vi "PrintLabel.vi"(6 "Print":bool, 7 "printer name (default)":string, 8 "Fixture_Data":u16[](array[numeric]), 11 "OPC_Model Type":u16 format="%x") -> ()   [LabVIEW 2017]
uses:
  <vilib>/Utility/NIReport.llb/Append Report Text (str wrap).vi
  <vilib>/Utility/NIReport.llb/NI_report.lvclass
panel:
  out "Even 2.5":string=" RR         "
  out "Line":string="KB E127652 191121SD1 0123 17:25"
  in  "margins (1.00)":T1={"top"=0.15, "left"=0.01, "right"=0.001, "bottom"=0.001} {"right" format="%.2f"; "bottom" format="%.2f"; "top" format="%.2f"; "left" format="%.2f"}
  out "Header":string="KB E127652 191121SD1 0123 17:25"
  out "Even 1.1":string=">MEGA     "
  out "Even 1.2":string=">PAD        "
  out "Even 1.3":string=" PIN       "
  out "Even 1.4":string=" WDW       "
  out "Even 1.5":string=" DL            "
  out "Even 2.1":string=" FR         "
  out "Even 2.2":string=">FL           "
  out "Even 2.3":string=">RL           "
  out "Even 2.4":string=" RR         "
  # "00 Product Number"
  # "10 Lane Number"
  # "20 Laser Number"
  # "21 Laser Number"
  # "30 Fixture Result"
  # "40 Master Unit"
  # "60 Mega Test"
  # "70 Windows Lock Press"
  # "71 Windows Lock Unpress"
  # "80 Door Lock"
  # "81 Door Unlock"
  # "90 FR Man Up"
  # "91 FR Man Down"
  # "92 FR Auto Up"
  # "93 FR Auto Down"
  # "100 RR Man Up"
  # "101 RR Man Down"
  # "110 FL Man Up"
  # "111 FL Man Down"
  # "112 FL Auto Up"
  # "113 FL  Down"
  # "120 RL Man Up"
  # "121 RL Man Down"
  # "130 LIN DR Up Contact"
  # "131 LIN DR Down Contact"
  # "132 LIN DR Auto Status"
  # "133 LIN AS Up Contact"
  # "134 LIN AS Down Contact"
  # "135 LIN AS Auto Status"
  # "136 WDW Lock Status"
  # "140 Vision Illumination"
  # "150 Vision Pin"
  # "160 QR Code Reader"
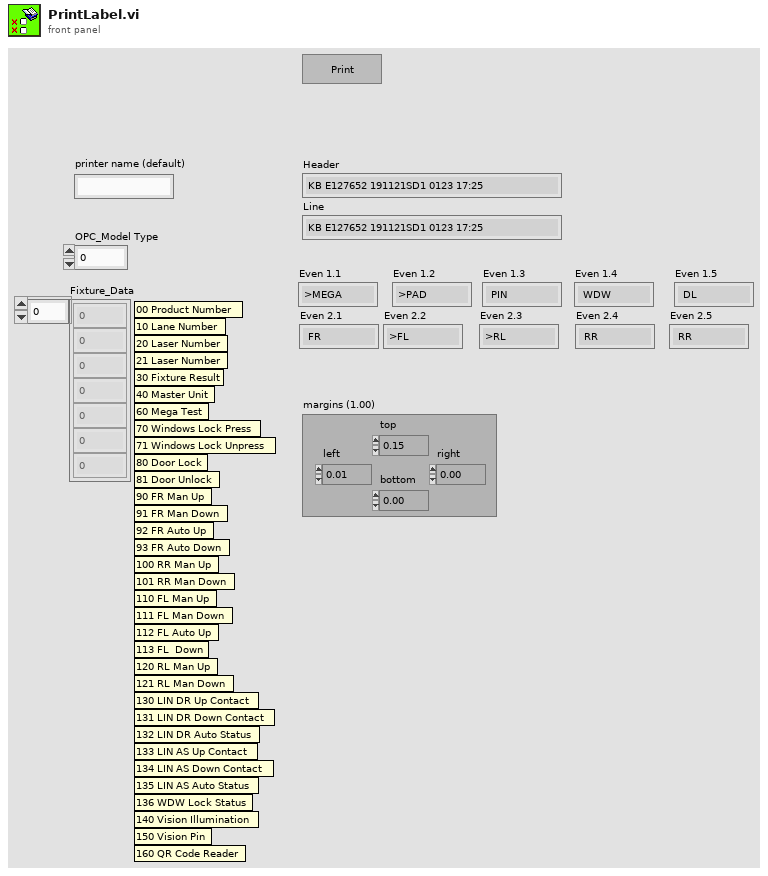
[diagram p1: front panel]
types:
  T1 = cluster{"top":dbl, "left":dbl, "right":dbl, "bottom":dbl}
  T2 = cluster{"Italic":enum16{"Italic Unchanged", "Italic On", "Italic Off"}, "Strike Through":enum16{"Strike Through Unchanged", "Strike Through On", "Strike Through Off"}, "Underline":enum16{"Underline Unchanged", "Underline On", "Underline Off"}, "Bold":enum16{"Bold Unchanged", "Bold On", "Bold Off"}}
  T3 = cluster{"Charset (-1)":i16, "Weight (-1)":i16, "Name":string, "Size":string}
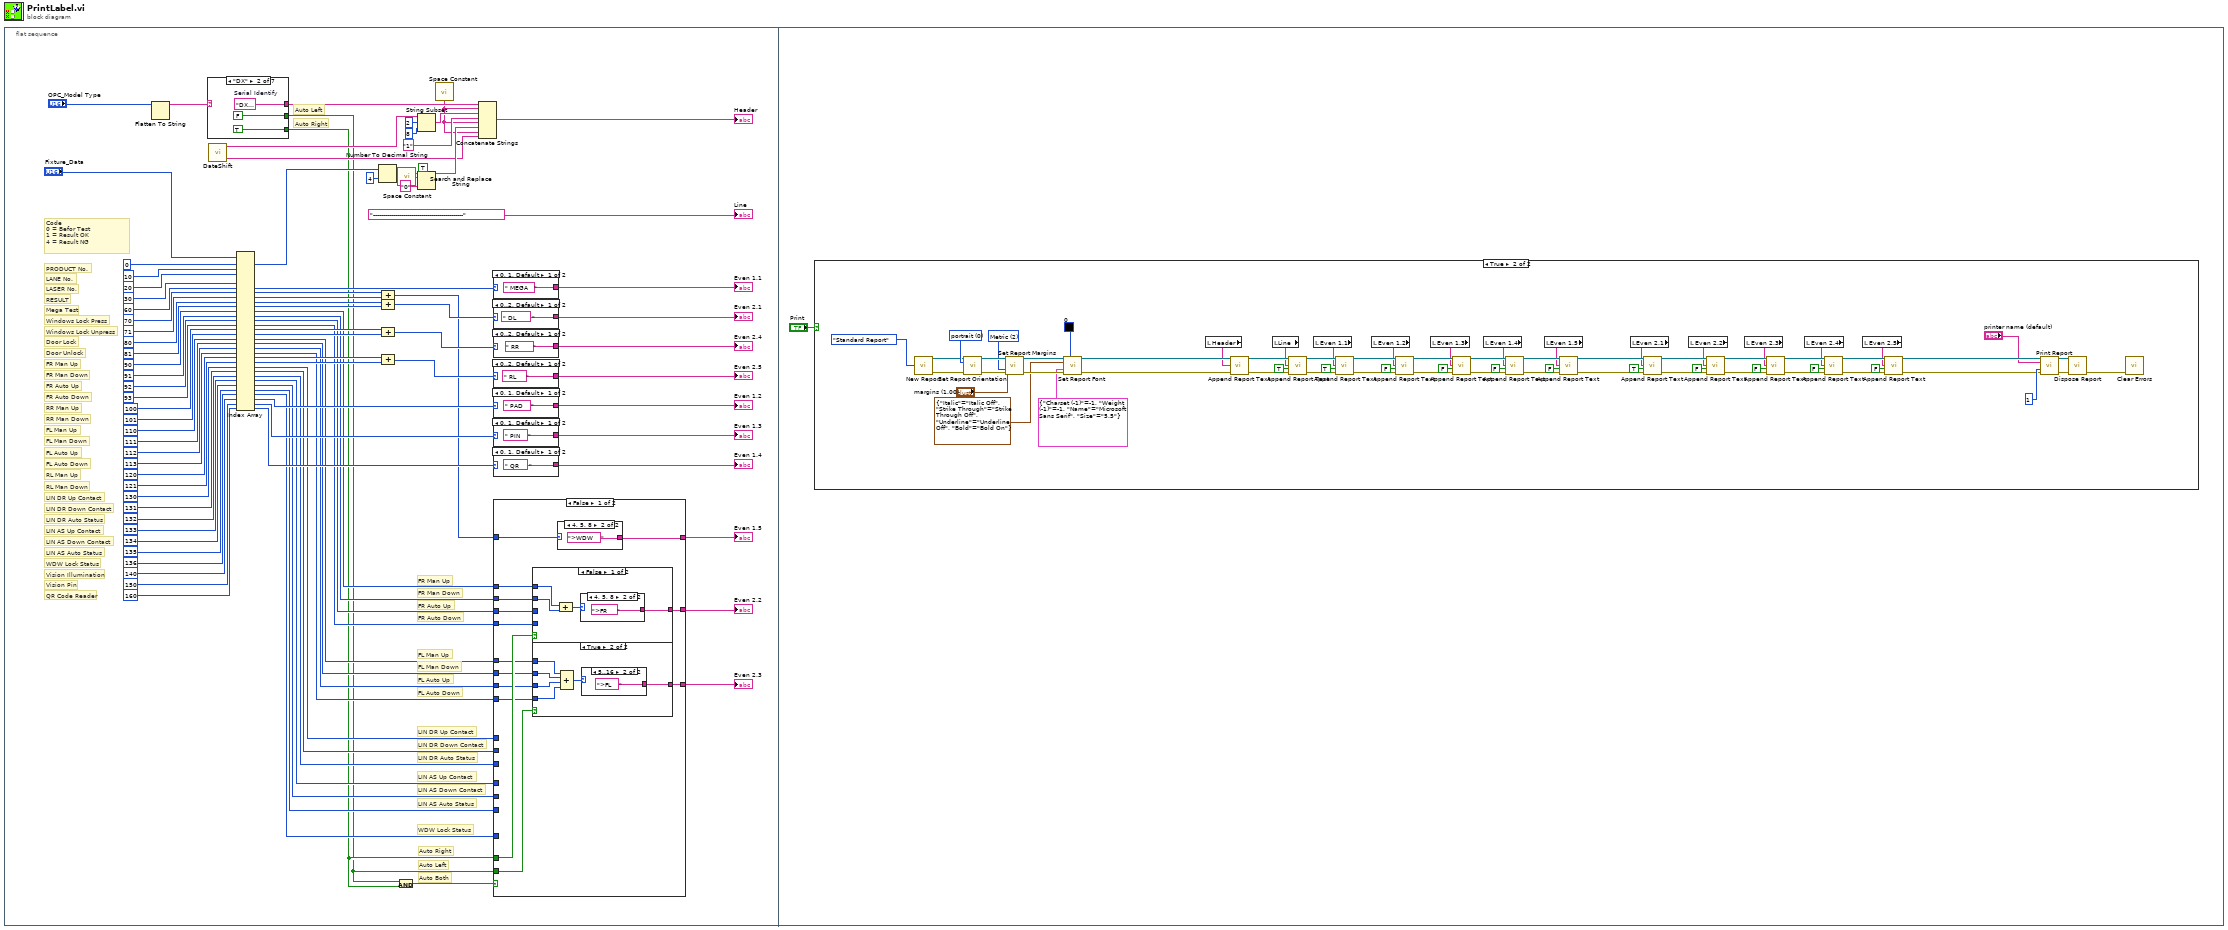
[diagram p0: block diagram]
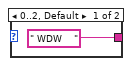
[diagram p2: hidden frame]
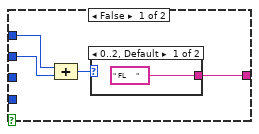
[diagram p3: hidden frame]
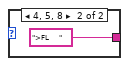
[diagram p4: hidden frame]
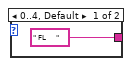
[diagram p5: hidden frame]
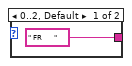
[diagram p6: hidden frame]
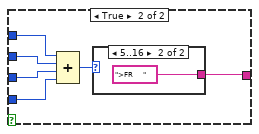
[diagram p7: hidden frame]
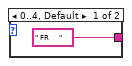
[diagram p8: hidden frame]
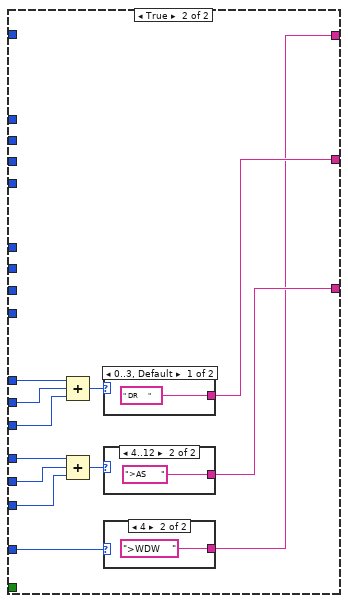
[diagram p9: hidden frame]
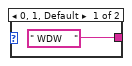
[diagram p10: hidden frame]
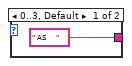
[diagram p11: hidden frame]
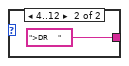
[diagram p12: hidden frame]
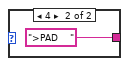
[diagram p13: hidden frame]
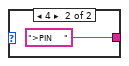
[diagram p14: hidden frame]
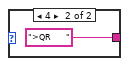
[diagram p15: hidden frame]
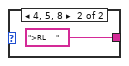
[diagram p16: hidden frame]
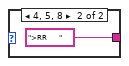
[diagram p17: hidden frame]
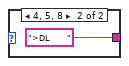
[diagram p18: hidden frame]
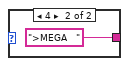
[diagram p19: hidden frame]
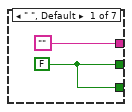
[diagram p20: hidden frame]
diagram:
  n1 = flat-sequence {
    frame #0 {
      # "Auto Right"
      # "Auto Left"
      # "FL Auto Down"
      # "FL Auto Up"
      # "FL Man Down"
      # "FL Man Up"
      # "FR Auto Down"
      # "FR Auto Up"
      # "FR Man Down"
      # "FR Man Up"
      # "WDW Lock Status"
      # "LIN AS Auto Status"
      # "LIN AS Down Contact"
      # "LIN AS Up Contact"
      # "LIN DR Auto Status"
      # "LIN DR Down Contact"
      # "LIN DR Up Contact"
      # "Auto Both"
      # "Auto Left"
      # "Auto Right"
      # "Code\n0 = Befor Test\n1 = Result OK\n4 = Result NG"
      # "LASER No."
      # "RESULT"
      # "LANE No."
      # "PRODUCT No."
      # "WDW Lock Status"
      # "QR Code Reader"
      # "Vision Pin"
      # "Vision Illumination"
      # "LIN AS Auto Status"
      # "LIN AS Down Contact"
      # "LIN AS Up Contact"
      # "LIN DR Auto Status"
      # "LIN DR Down Contact"
      # "LIN DR Up Contact"
      # "RL Man Down"
      # "RL Man Up"
      # "FL Auto Down"
      # "FL Auto Up"
      # "FL Man Down"
      # "FL Man Up"
      # "RR Man Down"
      # "RR Man Up"
      # "FR Auto Down"
      # "FR Auto Up"
      # "FR Man Down"
      # "FR Man Up"
      # "Door Unlock"
      # "Door Lock"
      # "Windows Lock Unpress"
      # "Windows Lock Press"
      # "Mega Test"
      n2 = Flatten To String(anything="OPC_Model Type") -> (data string=w62:string)  [unwired: 3 in, 2 out]
      n3 = case shown="\"DX\"" w62 {
        tunnel: ["" w176 w179 w182 w185 w188 w191] -> w61
        tunnel: [w172 FALSE TRUE TRUE FALSE TRUE TRUE] -> w1
        tunnel: [w172 TRUE TRUE TRUE TRUE FALSE FALSE] -> w2
        frame " ", Default {
          w172 = FALSE
        }
        frame "DX" {
          w176 = "DX E173839"  # Serial Identify
        }
        frame "K3" {
          w179 = "K3 E151441"  # Serial Identify
        }
        frame "4U" {
          w182 = "4U E148761"  # Serial Identify
        }
        frame "WS" {
          w185 = "WS E132857"  # Serial Identify
        }
        frame "L5" {
          w188 = "L5 E158515"  # Serial Identify
        }
        frame "KB" {
          w191 = "KB E127652"  # Serial Identify
        }
      }
      n4 = call "DateShift.vi"() -> ("RealTime"=w47:string, "DateShift"=w56:string)  [unwired: 3 in, 1 out]
      n5 = Index Array(array="Fixture_Data", index #1=0 ("index"), index #2=10 ("index"), index #3=20 ("index"), index #5=30 ("index"), index #6=60 ("index"), index #7=70 ("index"), index #8=71 ("index"), index #9=80 ("index"), index #10=81 ("index"), index #11=90 ("index"), index #12=91 ("index"), index #13=92 ("index"), index #14=93 ("index"), index #15=100 ("index"), index #16=101 ("index"), index #17=110 ("index"), index #18=111 ("index"), index #19=112 ("index"), index #20=113 ("index"), index #21=120 ("index"), index #22=121 ("index"), index #23=130 ("index"), index #24=131 ("index"), index #25=132 ("index"), index #26=133 ("index"), index #27=134 ("index"), index #28=135 ("index"), index #29=136 ("index"), index #30=140 ("index"), index #31=150 ("index"), index #32=160 ("index")) -> (element #1=w50:u16, element #6=w46:u16, element #7=w45:u16, element #8=w44:u16, element #9=w43:u16, element #10=w42:u16, element #11=w15:u16, element #12=w16:u16, element #13=w17:u16, element #14=w18:u16, element #15=w40:u16, element #16=w39:u16, element #17=w19:u16, element #18=w20:u16, element #19=w21:u16, element #20=w22:u16, element #21=w38:u16, element #22=w37:u16, element #23=w23:u16, element #24=w24:u16, element #25=w25:u16, element #26=w26:u16, element #27=w27:u16, element #28=w28:u16, element #29=w29:u16, element #30=w32:u16, element #31=w33:u16, element #32=w34:u16)  [unwired: 1 in, 4 out]
      n6 = Number To Decimal String(number=w50, width (-)=i16 4) -> (decimal integer string=w52:string)
      n7 = Compound Arithmetic op=ADD(w45, w44) -> (w30:u16)
      n8 = Compound Arithmetic op=ADD(w43, w42) -> (w41:u16)
      n9 = Compound Arithmetic op=ADD(w40, w39) -> (w36:u16)
      n10 = Compound Arithmetic op=ADD(w38, w37) -> (w35:u16)
      n11 = And(x=w1, y=w2) -> (x .and. y?=w31:bool)
      n12 = call <vilib>:"Space Constant.vi"() -> ("String"=w55:string)
      n13 = String Subset(string=w56, offset (0)=2, length (rest)=8 ("length (rest)")) -> (substring=w59:string)
      n14 = Search and Replace String(replace all?=TRUE ("replace all? (F)"), input string=w52, search string=w55, replace string="0" ("replace string (\"\")")) -> (result string=w49:string)  [unwired: 4 in, 3 out]
      n15 = call <vilib>:"Space Constant.vi"() -> ("String"=w48:string)
      n16 = Concatenate Strings(w61, w48, w59, "1" ("string"), w48, w49, w48, w47) -> (→"Header":string)
      n17 = case shown="0, 1, Default" w46 {
        tunnel: [" MEGA   " ">MEGA   "] -> w12
        frame 0, 1, Default {
        }
        frame 4 {
        }
      }
      "Even 1.1" <- w12
      n18 = case shown="0..2, Default" w41 {
        tunnel: [" DL        " ">DL      "] -> w11
        frame 0..2, Default {
        }
        frame 4, 5, 8 {
        }
      }
      "Even 2.1" <- w11
      n19 = case shown="0..2, Default" w36 {
        tunnel: [" RR       " ">RR      "] -> w10
        frame 0..2, Default {
        }
        frame 4, 5, 8 {
        }
      }
      "Even 2.4" <- w10
      n20 = case shown="0..2, Default" w35 {
        tunnel: [" RL     " ">RL     "] -> w9
        frame 0..2, Default {
        }
        frame 4, 5, 8 {
        }
      }
      "Even 2.5" <- w9
      n21 = case shown="0, 1, Default" w32 {
        tunnel: [" PAD    " ">PAD    "] -> w8
        frame 0, 1, Default {
        }
        frame 4 {
        }
      }
      "Even 1.2" <- w8
      n22 = case shown="0, 1, Default" w33 {
        tunnel: [" PIN    " ">PIN    "] -> w7
        frame 0, 1, Default {
        }
        frame 4 {
        }
      }
      "Even 1.3" <- w7
      n23 = case shown="0, 1, Default" w34 {
        tunnel: [" QR     " ">QR     "] -> w6
        frame 0, 1, Default {
        }
        frame 4 {
        }
      }
      "Even 1.4" <- w6
      n24 = case shown="False" w31 {
        tunnel: w1 -> [w98 _]
        tunnel: w2 -> [w105 _]
        tunnel: w30 -> [w97 _]
        tunnel: w29 -> [_ w141]
        tunnel: w28 -> [_ w143]
        tunnel: w27 -> [_ w144]
        tunnel: w26 -> [_ w145]
        tunnel: w25 -> [_ w148]
        tunnel: w24 -> [_ w149]
        tunnel: w23 -> [_ w150]
        tunnel: w22 -> [w100 _]
        tunnel: w21 -> [w101 _]
        tunnel: w20 -> [w102 _]
        tunnel: w19 -> [w103 _]
        tunnel: w18 -> [w106 _]
        tunnel: w17 -> [w107 _]
        tunnel: w16 -> [w108 _]
        tunnel: w15 -> [w109 _]
        tunnel: [w104 w147] -> w4
        tunnel: [w99 w142] -> w3
        tunnel: [w96 w140] -> w5
        frame False {
          n25 = case shown="False" w105 {
            tunnel: w109 -> [w129 w137]
            tunnel: w108 -> [w128 w136]
            tunnel: w107 -> [_ w135]
            tunnel: w106 -> [_ w134]
            tunnel: [w126 w132] -> w104
            frame False {
              n26 = Compound Arithmetic op=ADD(w129, w128) -> (w127:u16)
              n27 = case shown="4, 5, 8" w127 {
                tunnel: [" FR      " ">FR     "] -> w126
                frame 0..2, Default {
                }
                frame 4, 5, 8 {
                }
              }
            }
            frame True {
              n28 = Compound Arithmetic op=ADD(w137, w136, w135, w134) -> (w133:u16)
              n29 = case shown="5..16" w133 {
                tunnel: [" FR     " ">FR     "] -> w132
                frame 0..4, Default {
                }
                frame 5..16 {
                }
              }
            }
          }
          n30 = case shown="True" w98 {
            tunnel: w103 -> [w115 w123]
            tunnel: w102 -> [w114 w122]
            tunnel: w101 -> [_ w121]
            tunnel: w100 -> [_ w120]
            tunnel: [w112 w118] -> w99
            frame False {
              n31 = Compound Arithmetic op=ADD(w115, w114) -> (w113:u16)
              n32 = case shown="0..2, Default" w113 {
                tunnel: [" FL     " ">FL     "] -> w112
                frame 0..2, Default {
                }
                frame 4, 5, 8 {
                }
              }
            }
            frame True {
              n33 = Compound Arithmetic op=ADD(w123, w122, w121, w120) -> (w119:u16)
              n34 = case shown="5..16" w119 {
                tunnel: [" FL     " ">FL    "] -> w118
                frame 0..4, Default {
                }
                frame 5..16 {
                }
              }
            }
          }
          n35 = case shown="4, 5, 8" w97 {
            tunnel: [" WDW    " ">WDW    "] -> w96
            frame 0..2, Default {
            }
            frame 4, 5, 8 {
            }
          }
        }
        frame True {
          n36 = Compound Arithmetic op=ADD(w150, w149, w148) -> (w151:u16)
          n37 = Compound Arithmetic op=ADD(w145, w144, w143) -> (w146:u16)
          n38 = case shown="0..3, Default" w151 {
            tunnel: [" DR     " ">DR     "] -> w147
            frame 0..3, Default {
            }
            frame 4..12 {
            }
          }
          n39 = case shown="4..12" w146 {
            tunnel: [" AS     " ">AS     "] -> w142
            frame 0..3, Default {
            }
            frame 4..12 {
            }
          }
          n40 = case shown="4" w141 {
            tunnel: [" WDW    " ">WDW    "] -> w140
            frame 0, 1, Default {
            }
            frame 4 {
            }
          }
        }
      }
      "Even 1.5" <- w5
      "Even 2.2" <- w4
      "Even 2.3" <- w3
      "Line" <- "---------------------------------------------" ("text")
    }
    frame #1 {
      n41 = case shown="True" "Print" {
        frame False {
          n42 = Wait (ms)(milliseconds to wait=u32 250) -> ()  [unwired: 1 out]
        }
        frame True {
          w245 = u16 2 items=["Default", "US", "Metric"] ("measurement system (Default)")
          w259 = u16 0 items=["portrait", "landscape"] ("orientation (portrait)")
          n43 = call <vilib>:"New Report.vi"("report type"=enum16{"Standard Report", "HTML"}."Standard Report") -> ("report out"=w255:refnum<class "NI_report.lvclass">, "error out"=w256:errorcluster)  [unwired: 5 in, 8 out]
          n44 = call-dynamic "Set Report Orientation.vi"("report in"=w255, "orientation (portrait)"=w259, "error in (no error)"=w256) -> ("report out"=w258:refnum<class "NI_report.lvclass">, "error out"=w257:errorcluster)  [unwired: 11 out]
          n45 = call-dynamic "Set Report Margins.vi"("report in"=w258, "margins (1.00)"="margins (1.00)", "measurement system (default)"=w245, "error in (no error)"=w257) -> ("report out"=w253:refnum<class "NI_report.lvclass">, "error out"=w252:errorcluster)  [unwired: 10 out]
          n46 = call-dynamic "Set Report Font.vi"("report in"=w253, "text color (unchanged)"=u32 0, "text options"=T2 {"Italic"=enum."Italic Off", "Strike Through"=enum."Strike Through Off", "Underline"=enum."Underline Off", "Bold"=enum."Bold On"}, "font settings"=T3 {"Charset (-1)"=-1, "Weight (-1)"=-1, "Name"="Microsoft Sans Serif", "Size"="5.5"}, "error in (no error)"=w252) -> ("report out"=w244:refnum<class "NI_report.lvclass">, "error out"=w243:errorcluster)  [unwired: 8 in, 1 out]
          n47 = local read "Header"() -> (w205:string)
          n48 = call-poly <vilib>:"Append Report Text.vi"("report in"=w244, "text"=w205, "error in (no error)"=w243) -> ("report out"=w242:refnum<class "NI_report.lvclass">, "error out"=w241:errorcluster)  [unwired: 9 in, 2 out]
          n49 = local read "Line"() -> (w204:string)
          n50 = call-poly <vilib>:"Append Report Text.vi"("report in"=w242, "text"=w204, "append on new line? (F)"=TRUE, "error in (no error)"=w241) -> ("report out"=w239:refnum<class "NI_report.lvclass">, "error out"=w238:errorcluster)  [unwired: 8 in, 2 out]
          n51 = local read "Even 1.1"() -> (w203:string)
          n52 = call-poly <vilib>:"Append Report Text.vi"("report in"=w239, "text"=w203, "append on new line? (F)"=TRUE, "error in (no error)"=w238) -> ("report out"=w236:refnum<class "NI_report.lvclass">, "error out"=w235:errorcluster)  [unwired: 8 in, 2 out]
          n53 = local read "Even 1.2"() -> (w202:string)
          n54 = call-poly <vilib>:"Append Report Text.vi"("report in"=w236, "text"=w202, "append on new line? (F)"=FALSE, "error in (no error)"=w235) -> ("report out"=w233:refnum<class "NI_report.lvclass">, "error out"=w232:errorcluster)  [unwired: 8 in, 2 out]
          n55 = local read "Even 1.3"() -> (w201:string)
          n56 = call-poly <vilib>:"Append Report Text.vi"("report in"=w233, "text"=w201, "append on new line? (F)"=FALSE, "error in (no error)"=w232) -> ("report out"=w223:refnum<class "NI_report.lvclass">, "error out"=w222:errorcluster)  [unwired: 8 in, 2 out]
          n57 = local read "Even 1.4"() -> (w200:string)
          n58 = call-poly <vilib>:"Append Report Text.vi"("report in"=w223, "text"=w200, "append on new line? (F)"=FALSE, "error in (no error)"=w222) -> ("report out"=w225:refnum<class "NI_report.lvclass">, "error out"=w226:errorcluster)  [unwired: 8 in, 2 out]
          n59 = local read "Even 1.5"() -> (w199:string)
          n60 = call-poly <vilib>:"Append Report Text.vi"("report in"=w225, "text"=w199, "append on new line? (F)"=FALSE, "error in (no error)"=w226) -> ("report out"=w228:refnum<class "NI_report.lvclass">, "error out"=w229:errorcluster)  [unwired: 8 in, 2 out]
          n61 = local read "Even 2.1"() -> (w198:string)
          n62 = call-poly <vilib>:"Append Report Text.vi"("report in"=w228, "text"=w198, "append on new line? (F)"=TRUE, "error in (no error)"=w229) -> ("report out"=w214:refnum<class "NI_report.lvclass">, "error out"=w213:errorcluster)  [unwired: 8 in, 2 out]
          n63 = local read "Even 2.2"() -> (w197:string)
          n64 = call-poly <vilib>:"Append Report Text.vi"("report in"=w214, "text"=w197, "append on new line? (F)"=FALSE, "error in (no error)"=w213) -> ("report out"=w220:refnum<class "NI_report.lvclass">, "error out"=w219:errorcluster)  [unwired: 8 in, 2 out]
          n65 = local read "Even 2.3"() -> (w196:string)
          n66 = call-poly <vilib>:"Append Report Text.vi"("report in"=w220, "text"=w196, "append on new line? (F)"=FALSE, "error in (no error)"=w219) -> ("report out"=w217:refnum<class "NI_report.lvclass">, "error out"=w216:errorcluster)  [unwired: 8 in, 2 out]
          n67 = local read "Even 2.4"() -> (w195:string)
          n68 = call-poly <vilib>:"Append Report Text.vi"("report in"=w217, "text"=w195, "append on new line? (F)"=FALSE, "error in (no error)"=w216) -> ("report out"=w211:refnum<class "NI_report.lvclass">, "error out"=w210:errorcluster)  [unwired: 8 in, 2 out]
          n69 = local read "Even 2.5"() -> (w194:string)
          n70 = call-poly <vilib>:"Append Report Text.vi"("report in"=w211, "text"=w194, "append on new line? (F)"=FALSE, "error in (no error)"=w210) -> ("report out"=w209:refnum<class "NI_report.lvclass">, "error out"=w208:errorcluster)  [unwired: 8 in, 2 out]
          n71 = call-dynamic "Print Report.vi"("report in"=w209, "printer name (default)"="printer name (default)", "number of copies (1)"=1, "error in (no error)"=w208) -> ("report out"=w248:refnum<class "NI_report.lvclass">, "error out"=w247:errorcluster)  [unwired: 10 in]
          n72 = call-dynamic "Dispose Report.vi"("report in"=w248, "error in (no error)"=w247) -> ("error out"=w207:errorcluster)  [unwired: 3 in, 10 out]
          n73 = call <vilib>:"Clear Errors.vi"("error in (no error)"=w207) -> ()  [unwired: 5 in, 2 out]
        }
      }
    }
  }
